vi "Add Items.vi"() -> ()   [LabVIEW 2018, in "OPC UA.lvlib"]
uses:
  OPC UA.lvlib
  <vilib>/OPCUA/controls/Data Type.ctl
  <vilib>/OPCUA/controls/NodeId.ctl
  <vilib>/OPCUA/server/Add Dialog Condition.vi
  <vilib>/OPCUA/NI OPC UA Server.lvlib
panel:
  out "error out":errorcluster
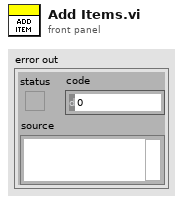
[diagram p1: front panel]
types:
  T1 = typedef "Data Type.ctl" = u16
  T2 = cluster{"name":string, "data type":T1, "access level":u16, "description":string}
  T3 = typedef "NodeId.ctl" = string
  T4 = cluster{"condition name":string, "source node ID":T3, "prompt":string, "description":string}
  T5 = typedef "OPC UA Server Refnum.ctl" = refnum<k21>
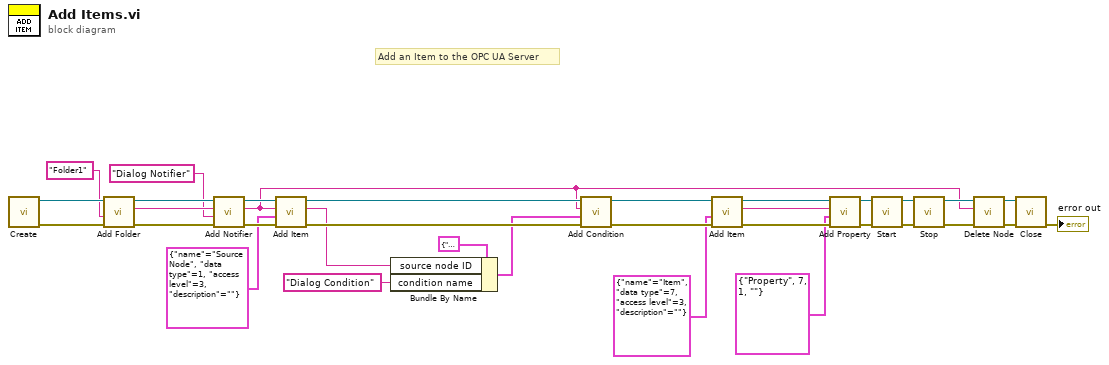
[diagram p0: block diagram]
diagram:
  # "Add an Item to the OPC UA Server"
  n1 = call <vilib>:"Create.vi"() -> ("error out"=w32:errorcluster, "OPC UA server refnum out"=w33:T5)  [unwired: 9 in, 1 out]
  n2 = call <vilib>:"Add Folder.vi"("error in (no error)"=w32, "folder name"="Folder1", "OPC UA server refnum in"=w33) -> ("error out"=w31:errorcluster, "folder node ID"=w15:T3, "OPC UA server refnum out"=w23:T5)  [unwired: 5 in]
  n3 = call <vilib>:"Add Notifier.vi"("error in (no error)"=w31, "notifier name"="Dialog Notifier", "parent folder node ID"=w15, "OPC UA server refnum in"=w23) -> ("error out"=w30:errorcluster, "notifier node ID"=w4:T3, "OPC UA server refnum out"=w22:T5)  [unwired: 3 in, 1 out]
  n4 = call <vilib>:"Add Item.vi"("error in (no error)"=w30, "item"=T2 {"name"="Source Node", "data type"=1, "access level"=3, "description"=""}, "parent folder node ID"=w4, "OPC UA server refnum in"=w22) -> ("error out"=w29:errorcluster, "item node ID"=w7:T3, "OPC UA server refnum out"=w21:T5)  [unwired: 3 in, 1 out]
  n5 = Bundle By Name(cluster=T4 {"condition name"="", "source node ID"="", "prompt"="", "description"=""} ("property"), "source node ID"=w7, "condition name"="Dialog Condition") -> (w5:T4)
  n6 = call-poly <vilib>:"Add Condition.vi"("error in (no error)"=w29, "property"=w5, "notifier node ID"=w4, "OPC UA server refnum in"=w21) -> ("error out"=w28:errorcluster, "OPC UA server refnum out"=w20:T5)  [unwired: 4 in, 2 out]
  n7 = call <vilib>:"Add Item.vi"("error in (no error)"=w28, "item"=T2 {"name"="Item", "data type"=7, "access level"=3, "description"=""}, "OPC UA server refnum in"=w20) -> ("error out"=w27:errorcluster, "item node ID"=w3:T3, "OPC UA server refnum out"=w19:T5)  [unwired: 4 in, 1 out]
  n8 = call <vilib>:"Add Property.vi"("error in (no error)"=w27, "property"=T2 {"name"="Property", "data type"=7, "access level"=1, "description"=""}, "item node ID"=w3, "OPC UA server refnum in"=w19) -> ("error out"=w26:errorcluster, "OPC UA server refnum out"=w18:T5)  [unwired: 3 in, 2 out]
  n9 = call <vilib>:"Start.vi"("error in (no error)"=w26, "OPC UA server refnum in"=w18) -> ("error out"=w25:errorcluster, "OPC UA server refnum out"=w17:T5)  [unwired: 7 in, 1 out]
  n10 = call <vilib>:"Stop.vi"("error in (no error)"=w25, "OPC UA server refnum in"=w17) -> ("error out"=w13:errorcluster, "OPC UA server refnum out"=w10:T5)  [unwired: 8 in]
  n11 = call <vilib>:"Delete Node.vi"("error in (no error)"=w13, "node ID"=w4, "OPC UA server refnum in"=w10) -> ("error out"=w12:errorcluster, "OPC UA server refnum out"=w11:T5)  [unwired: 7 in]
  n12 = call <vilib>:"Close.vi"("error in (no error)"=w12, "OPC UA server refnum in"=w11) -> ("error out"=→"error out":errorcluster)  [unwired: 9 in]
